vi "run.update.endtime.vi"(8 "error in":errorcluster, 9 "End (now)":timestamp format="%<%x %.3X>T", 10 "Run":refnum<class "Run.lvclass">, 11 "Nominal Client in":refnum<class "Nominal Client.lvclass">) -> (0 "error out":errorcluster, 2 "Run out":refnum<class "Run.lvclass">, 3 "Nominal Client out":refnum<class "Nominal Client.lvclass">)   [LabVIEW 2020]
doc: "Create a new run in Nominal.\nThrows if start is equal to or after end."
uses:
  Nominal Client.lvclass
  Run/Run.lvclass
  Run/Run.lvclass/Run.ctl
  Run/rid.get.vi
  Nominal Client.lvclass/Nominal Client.ctl
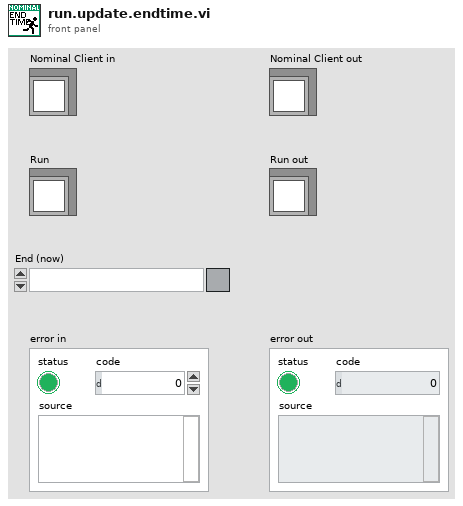
[diagram p1: front panel]
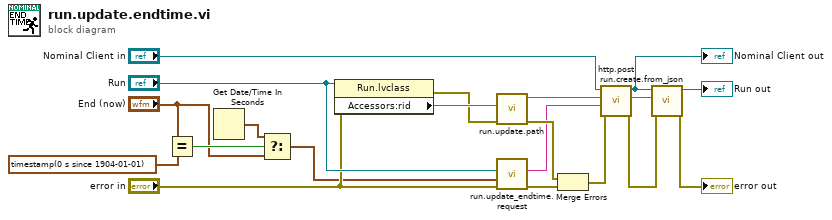
[diagram p0: block diagram]
diagram:
  n1 = Equal?(x="End (now)", y=timestamp(0 s since 1904-01-01) ("End (now)")) -> (x = y?=w5:bool)
  n2 = Get Date/Time In Seconds() -> (seconds since 1Jan1904=w3:timestamp)
  n3 = Select(t=w3, s=w5, f="End (now)") -> (s? t:f=w2:timestamp)
  n4 = property class="Run.lvclass"(reference="Run", error in="error in") -> (error out=w14:errorcluster, "Accessors:rid"=w16:string)  [unwired: 1 out]
  n5 = call "run.update.path.vi"("error in"=w14, "rid"=w16) -> ("error out"=w13:errorcluster, "path"=w15:string)  [unwired: 8 in]
  n6 = call "run.update_endtime.request.vi"("error in (no error)"="error in", "End"=w2, "Run"="Run") -> ("error out"=w8:errorcluster, "Request Body"=w7:string)  [unwired: 7 in]
  n7 = Merge Errors(w13, w8) -> (w17:errorcluster)
  n8 = call "http.post.vi"("error in"=w17, "Request body"=w7, "Path"=w15, "Nominal Client in"="Nominal Client in") -> ("error out"=w19:errorcluster, "Response"=w20:string, "Nominal Client out"=w1:refnum<class "Nominal Client.lvclass">)  [unwired: 4 in, 1 out]
  "Nominal Client out" <- w1
  n9 = call "run.create.from_json.vi"("error in"=w19, "JSON"=w20, "Nominal Client"=w1) -> ("error out"=→"error out":errorcluster, "Run out"=→"Run out":refnum<class "Run.lvclass">)  [unwired: 7 in]
